vi "AutoSetUpMetodo.vi"(8 "error in (no error)":errorcluster, 11 "Keysight in":refnum<class "Edu-1200.lvclass">) -> (0 "error out":errorcluster, 3 "Keysight out":refnum<class "Edu-1200.lvclass">)   [LabVIEW 2020, in "Edu-1200.lvclass"]
uses:
  Edu-1200.lvclass
  Edu-1200.lvclass/Edu-1200.ctl
  <instrlib>/Agilent 2000 3000 X-Series/Agilent 2000 3000 X-Series.lvlib
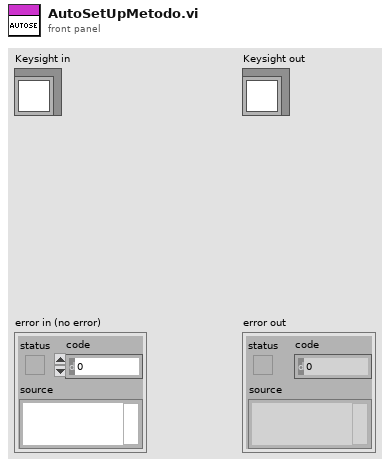
[diagram p1: front panel]
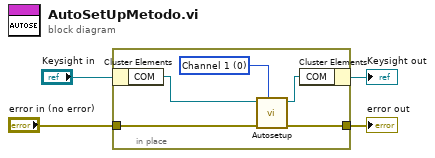
[diagram p0: block diagram]
diagram:
  n1 = in-place {
    in-place-border: "error in (no error)" -> [w7]
    in-place-border: [w6] -> w1
    w5 = 0 items=["Channel 1"=0, "Channel 2"=1, "Channel 3"=2, "Channel 4"=3, "Digital Bus Low"=9, "Digital Bus High"=10] ("Auto Scale Source (0: Channel 1)")
    n2 = in-place-cluster #1("Keysight in") -> ("COM"=w9:refnum<visa-resource-name>)
    n3 = call <instrlib>:"Autosetup.vi"("Auto Scale Source (0: Channel 1)"=w5, "error in (no error)"=w7, "VISA resource name"=w9) -> ("error out"=w6:errorcluster, "VISA resource name out"=w8:refnum<visa-resource-name>)  [unwired: 7 in]
    n4 = in-place-cluster #1("COM"=w8) -> (→"Keysight out":refnum<class "Edu-1200.lvclass">)
  }
  "error out" <- w1
